vi "XML - Remove Old Rx Channels.vi"(8 "error in (no error)":errorcluster, 11 "Device Item Ref in":T1 format="%.0x") -> (0 "error out":errorcluster, 2 "Rx Dependent Refs":T1[](array[typedef]) format="%.0x", 3 "Device Item Ref out":T1 format="%.0x")   [LabVIEW 2019]
uses:
  <vilib>/NI VeriStand/Custom Device API/Custom Device Item Ref.ctl
  Shared/Constants.vi
  <vilib>/NI VeriStand/Custom Device Tools/Custom Device Utility Library/NI VeriStand - Search for Item by GUID.vi
  <vilib>/NI VeriStand/Custom Device Tools/Custom Device Utility Library/Custom Device Utility Library.lvlib
  <vilib>/NI VeriStand/Custom Device API/Custom Device API.lvlib
  Shared/UDP-Custom-Device Shared.lvlib
  Property Accessors/Shared Packet Accessors.lvlib
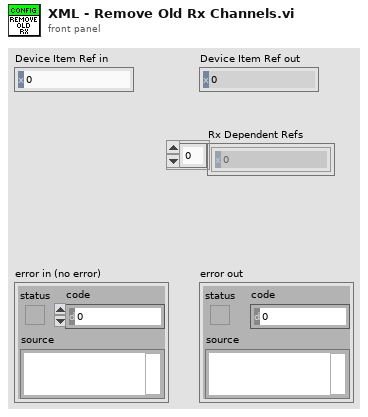
[diagram p1: front panel]
types:
  T1 = typedef "Custom Device API.lvlib/Custom Device Item Ref.ctl" = u64
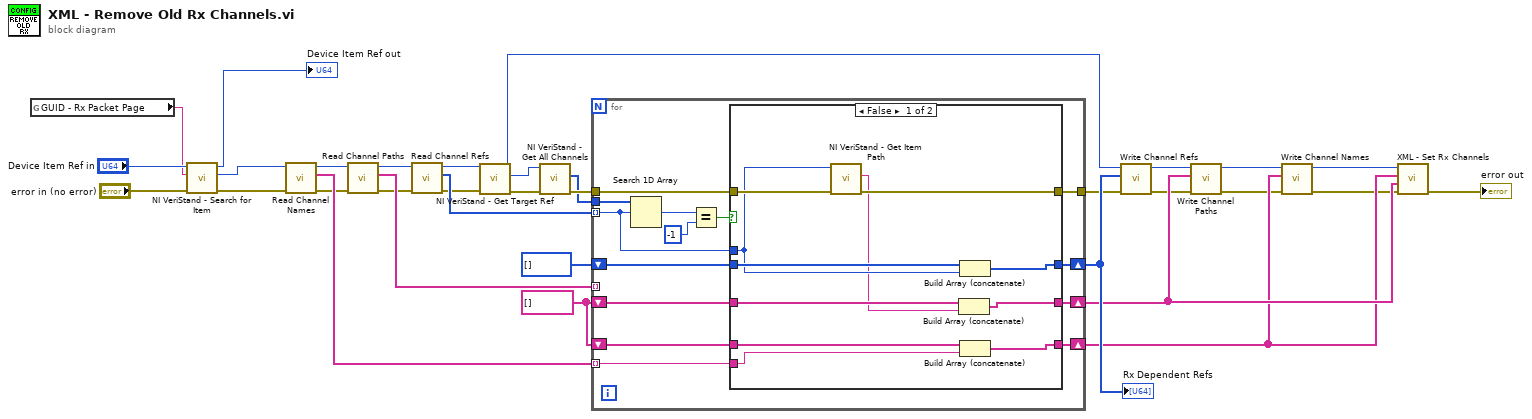
[diagram p0: block diagram]
diagram:
  w31 = string[] []
  n1 = global read "Constants.vi" "GUID - Rx Packet Page"() -> (w23:string)
  n2 = call-poly <vilib>:"NI VeriStand - Search for Item.vi"("error in"="error in (no error)", "Item GUID"=w23, "Section Ref in"="Device Item Ref in") -> ("error out"=w4:errorcluster, "Item Ref"=w16:T1, "Section Ref out"=→"Device Item Ref out":T1)  [unwired: 5 in, 1 out]
  n3 = call "Read Channel Names.vi"("error in (no error)"=w4, "Node Ptr"=w16) -> ("error out"=w5:errorcluster, "Channel Names"=w22:string[], "Node Ptr out"=w15:T1)  [unwired: 7 in]
  n4 = call "Read Channel Paths.vi"("error in (no error)"=w5, "Node Ptr"=w15) -> ("error out"=w6:errorcluster, "Channel Paths"=w21:string[], "Node Ptr out"=w14:T1)  [unwired: 7 in]
  n5 = call "Read Channel Refs.vi"("error in (no error)"=w6, "Node Ptr"=w14) -> ("error out"=w3:errorcluster, "Dependent Node Refs"=w20:T1[], "Node Ptr out"=w2:T1)  [unwired: 7 in]
  n6 = call <vilib>:"NI VeriStand - Get Target Ref.vi"("error in"=w3, "Item Ref in"=w2) -> ("error out"=w27:errorcluster, "Target Ref"=w28:T1, "Item Ref out"=w1:T1)  [unwired: 6 in, 1 out]
  n7 = call <vilib>:"NI VeriStand - Get All Channels.vi"("error in"=w27, "Section Ref in"=w28) -> ("error out"=w30:errorcluster, "Channel Refs"=w29:T1[])  [unwired: 6 in, 2 out]
  n8 = for {
    tunnel: w29 -> [w47]
    tunnel: w20 -> [w35] mode=indexing
    tunnel: w30 -> [w43]
    tunnel: w22 -> [w42] mode=indexing
    tunnel: w21 -> [_] mode=indexing
    shift-right: [w37] -> w18
    shift-left: w31 -> [w40]
    shift-right: [w36] -> w17
    shift-left: w31 -> [w41]
    shift-right: [w38] -> w19
    shift-left: T1[] [] -> [w39]
    tunnel: [w34] -> w7
    n9 = Search 1D Array(1D array=w47, element=w35) -> (index of element=w46:i32)  [unwired: 1 in]
    n10 = Equal?(x=w46, y=-1) -> (x = y?=w44:bool)
    n11 = case shown="False" w44 {
      tunnel: w43 -> [w51 w59]
      tunnel: w42 -> [w53 _]
      tunnel: w41 -> [w54 w60]
      tunnel: w40 -> [w56 w61]
      tunnel: w39 -> [w58 w62]
      tunnel: [w57 w62] -> w38
      tunnel: [w55 w61] -> w37
      tunnel: [w52 w60] -> w36
      tunnel: w35 -> [w50 _]
      tunnel: [w49 w59] -> w34
      frame False {
        n12 = call <vilib>:"NI VeriStand - Get Item Path.vi"("error in (no error)"=w51, "Item Ref in"=w50) -> ("error out"=w49:errorcluster, "Path"=w48:string)  [unwired: 6 in, 2 out]
        n13 = Build Array (concatenate)(w56, w48) -> (w55:string[])
        n14 = Build Array (concatenate)(w58, w50) -> (w57:T1[])
        n15 = Build Array (concatenate)(w54, w53) -> (w52:string[])
      }
      frame True {
      }
    }
  }
  "Rx Dependent Refs" <- w19
  n16 = call "Write Channel Refs.vi"("error in (no error)"=w7, "Dependent Node Refs"=w19, "Node Ptr"=w1) -> ("error out"=w9:errorcluster, "Node Ptr out"=w13:T1)  [unwired: 7 in]
  n17 = call "Write Channel Paths.vi"("error in (no error)"=w9, "Channel Paths"=w18, "Node Ptr"=w13) -> ("error out"=w8:errorcluster, "Node Ptr out"=w12:T1)  [unwired: 7 in]
  n18 = call "Write Channel Names.vi"("error in (no error)"=w8, "Channel Names"=w17, "Node Ptr"=w12) -> ("error out"=w10:errorcluster, "Node Ptr out"=w11:T1)  [unwired: 7 in]
  n19 = call "XML - Set Rx Channels.vi"("error in (no error)"=w10, "Rx Channel Paths"=w18, "Rx Channel Names"=w17, "Item Ref in"=w11) -> ("error out"=→"error out":errorcluster)  [unwired: 6 in, 1 out]
